vi "Read Rank.vi"(8 "error in (no error)":errorcluster, 11 "Scalar Path Group in":refnum<class "Scalar Path Group.lvclass">) -> (0 "error out":errorcluster, 2 "Rank":dbl, 3 "Scalar Path Group out":refnum<class "Scalar Path Group.lvclass">)   [LabVIEW 2023, in "RFFixtureCharact.Public.lvlib" / "Scalar Path Group.lvclass"]
uses:
  Scalar Path Group.lvclass
  Scalar Path Group.lvclass/Scalar Path Group.ctl
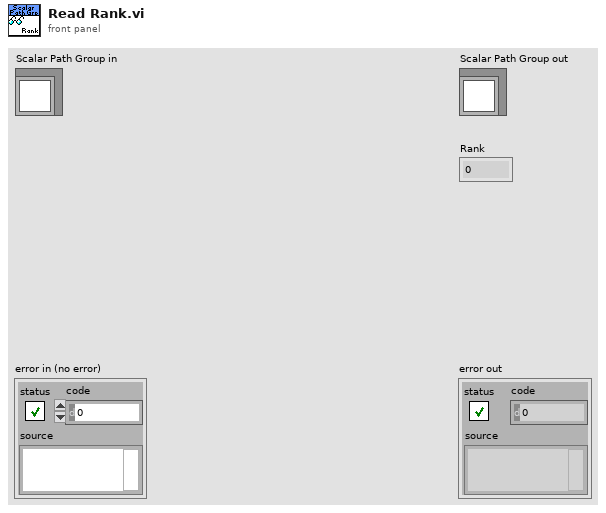
[diagram p1: front panel]
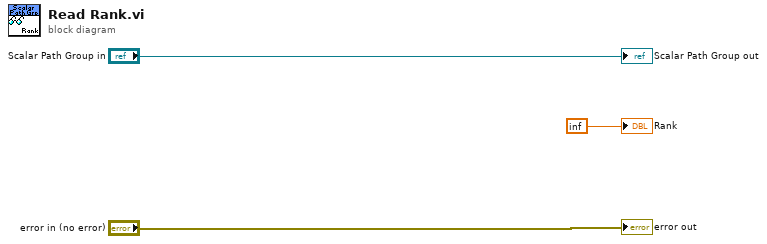
[diagram p0: block diagram]
diagram:
  "error out" <- "error in (no error)"
  "Scalar Path Group out" <- "Scalar Path Group in"
  "Rank" <- inf
